vi "Set GUI Parameters.vi"(0 "reference in":refnum<class "Generic Utilities.lvclass">, 5 "error in (no error)":errorcluster, 7 "GUI Parameters":T1) -> (14 "reference out":refnum<class "Generic Utilities.lvclass">, 19 "error out":errorcluster)   [LabVIEW 2020, in "Generic Utilities.lvclass"]
doc: "This will initalize the timer use for timing execution time."
uses:
  Generic Utilities.lvclass
  protected/GUI Parameters.ctl
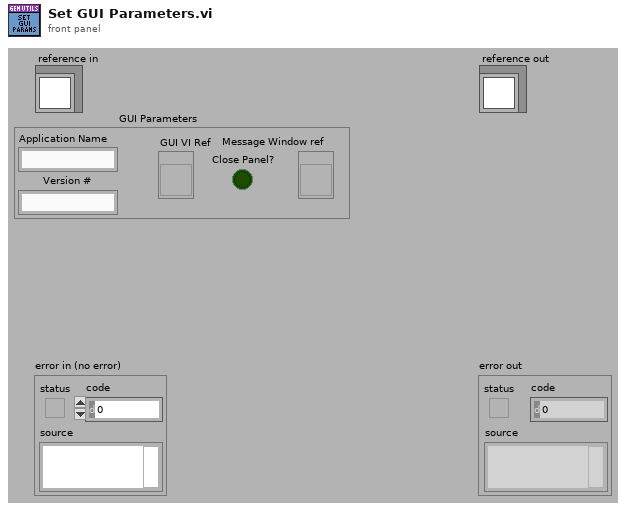
[diagram p1: front panel]
types:
  T1 = typedef "Generic Utilities.lvclass/GUI Parameters.ctl" = cluster{"Application Name":string, "GUI VI Ref":refnum<vi>, "Close Panel?":bool, "Message Window ref":refnum<vi>, "Version #":string}
  T2 = typedef "Generic Utilities.lvclass/ObjectAttributesRef.ctl" = refnum<data-value>
  T3 = typedef "Generic Utilities.lvclass/ObjectAttributes.ctl" = cluster{"GUI Parameters":T1, "State Machine Control":cluster{"Timeout":i32, "State Queue":string[], "State History":string[], "State History Length":i32}, "Logging File Path":path, "OBJ not a refnum?":bool, "Timer Start":timestamp, "FP Refnums":T4}
  T4 = typedef "Generic Utilities.lvclass/FP Refnums.ctl" = cluster{"Panel refnum":refnum<vi>, "Control Labels":string[], "Refnums":refnum<vi>[]}
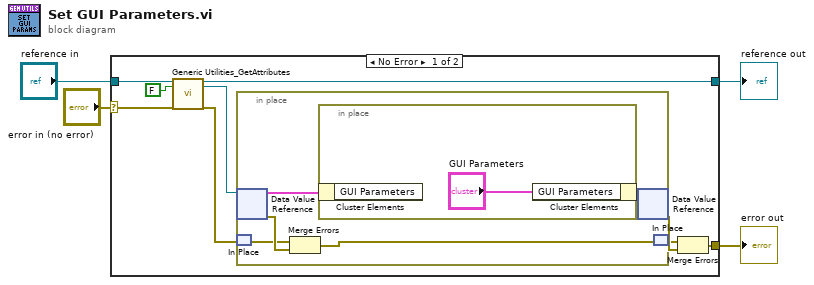
[diagram p0: block diagram]
diagram:
  n1 = case shown="No Error" "error in (no error)" {
    selector: "error in (no error)" -> [w9 w21]
    tunnel: [w13 w21] -> w3
    tunnel: [w8 w20] -> w1
    tunnel: "reference in" -> [w11 w20]
    frame No Error {
      n2 = call "Generic Utilities_GetAttributes.vi"("reference in"=w11, "return data? (T)"=FALSE, "error in (no error)"=w9) -> ("reference out"=w8:refnum<class "Generic Utilities.lvclass">, "attributes ref"=w7:T2, "error out"=w6:errorcluster)  [unwired: 13 in, 1 out]
      n3 = in-place {
        n4 = in-place-dvr #1(w7) -> (w17:T3, w16:errorcluster)
        n5 = in-place-match #2(w6) -> (w15:errorcluster)
        n6 = Merge Errors(w15, w16) -> (w14:errorcluster)
        n7 = in-place {
          n8 = in-place-cluster #3(w17) -> ()  [unwired: 1 out]
          n9 = in-place-cluster #3("GUI Parameters"="GUI Parameters") -> (w18:T3)
        }
        n10 = in-place-dvr #1(w18) -> (w12:errorcluster)  [unwired: 1 out]
        n11 = in-place-match #2(w14) -> (w5:errorcluster)
      }
      n12 = Merge Errors(w5, w12) -> (w13:errorcluster)
    }
    frame Error {
    }
  }
  "error out" <- w3
  "reference out" <- w1
